vi "Cluster_AURA.vi"(0 "FOTOCELULA":bool, 1 "RFID_Error":errorcluster, 4 "RFID_LR6_Error":errorcluster, 6 "DC":bool, 7 "TEMPERATURA":bool, 8 "WHEEL_SENSOR":bool, 9 "all rows":dbl[][](array[numeric]), 10 "LIMITE MAX":dbl, 11 "LIMITE MIN":dbl, 12 "ERROR FPGA":errorcluster, 13 "ERROR ESCRITURA":errorcluster) -> (20 "appended array":cluster{string, dbl, "output string":string}[](array[cluster]), 22 "ESTADO WRD":dbl)   [LabVIEW 2015]
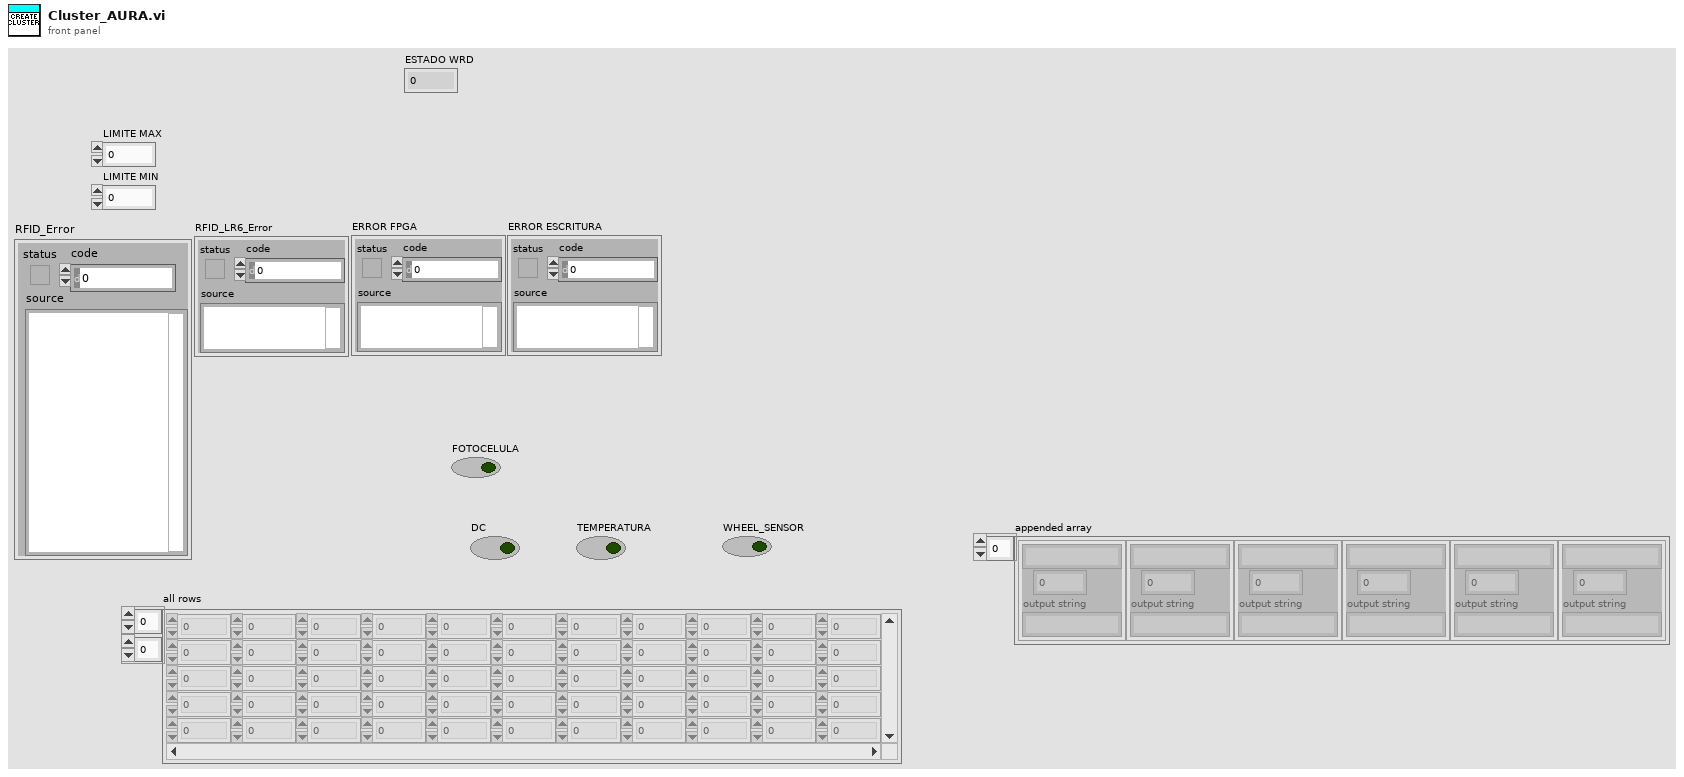
[diagram p1: front panel]
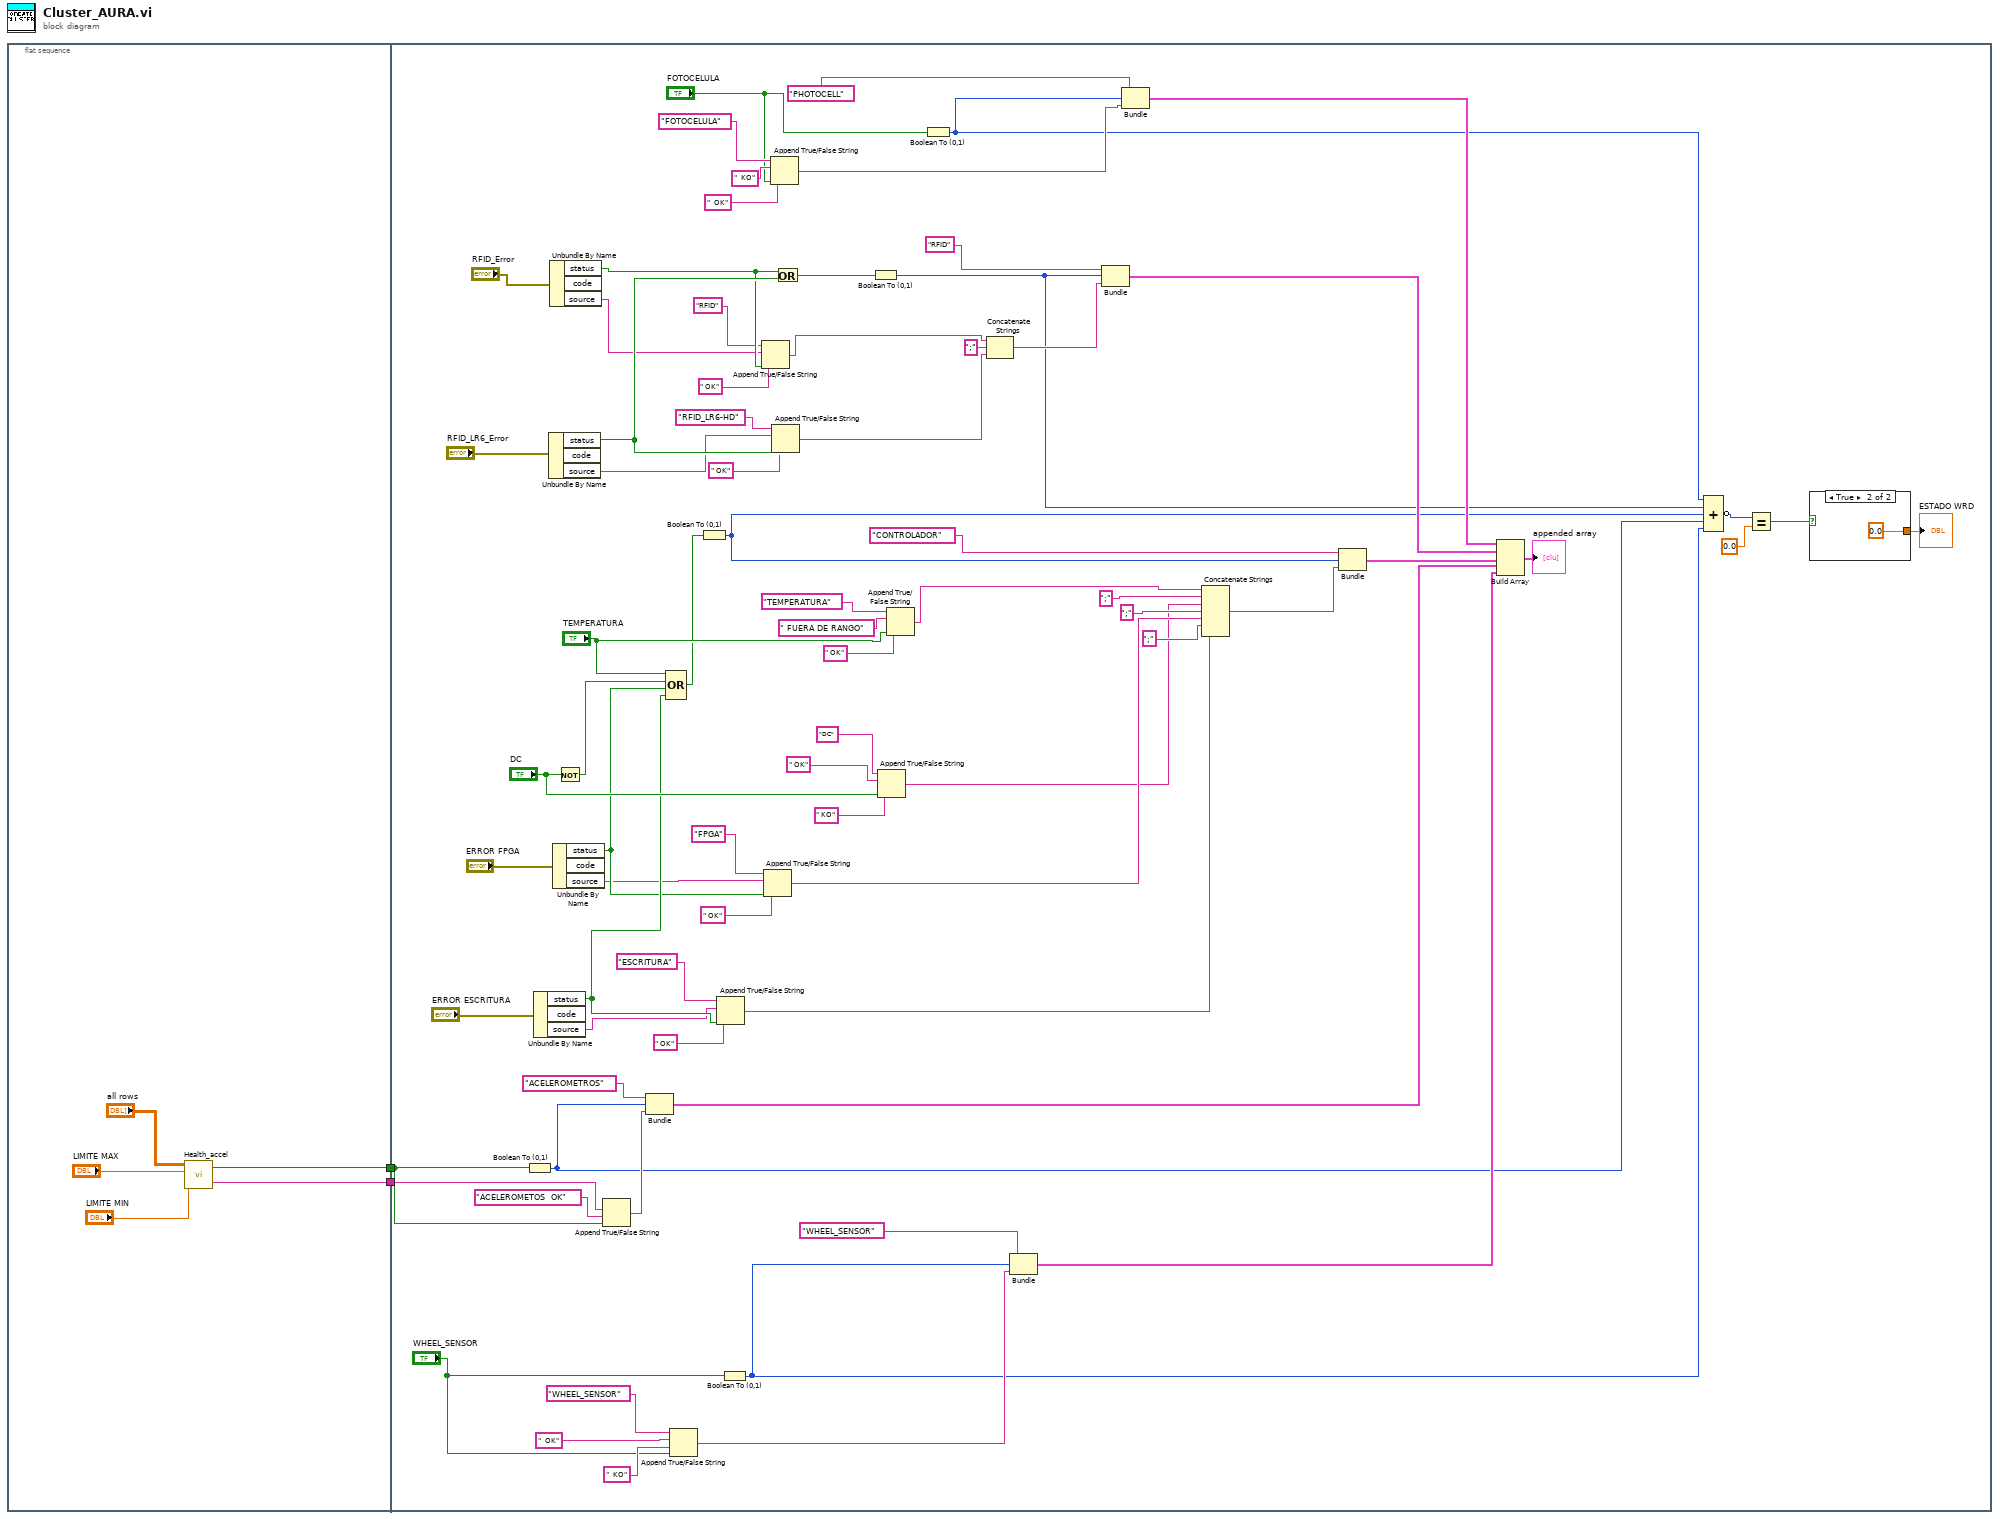
[diagram p0: block diagram]
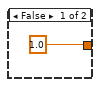
[diagram p2: hidden frame]
diagram:
  n1 = flat-sequence {
    tunnel: [w6] -> w2
    tunnel: [w5] -> w1
    tunnel: w2 -> [w31]
    tunnel: w1 -> [w11]
    frame #0 {
      n2 = call "Health_accel.vi"("LIMITE MIN"="LIMITE MIN", "LIMITE MAX"="LIMITE MAX", "Aceleraciones"="all rows") -> ("concatenated string"=w6:string, "ACELEROMETROS OK"=w5:bool)  [unwired: 3 in]
    }
    frame #1 {
      n3 = Boolean To (0,1)(Boolean=w11) -> (0, 1=w10:i16)
      n4 = Unbundle By Name("ERROR ESCRITURA") -> ("status"=w22:bool, "source"=w21:string)  [unwired: 1 out]
      n5 = Unbundle By Name("RFID_LR6_Error") -> ("status"=w72:bool, "source"=w26:string)  [unwired: 1 out]
      n6 = Unbundle By Name("RFID_Error") -> ("status"=w71:bool, "source"=w27:string)  [unwired: 1 out]
      n7 = Unbundle By Name("ERROR FPGA") -> ("status"=w19:bool, "source"=w18:string)  [unwired: 1 out]
      n8 = Not(x="DC") -> (.not. x?=w84:bool)
      n9 = Append True/False String(1:w11, 2:"ACELEROMETOS  OK" ("true string"), 3:w31) -> (0:w45:string)  [unwired: 1 in]
      n10 = Bundle("ACELEROMETROS", w10, "output string"=w45) -> (w51:cluster{string, i16, "output string":string})  [unwired: 1 in]
      n11 = Compound Arithmetic op=OR("TEMPERATURA", w84, w19, w22) -> (w13:bool)
      n12 = Append True/False String(1:"WHEEL_SENSOR", 2:"  KO" ("false string"), 3:"  OK" ("true string"), 4:"WHEEL_SENSOR" ("string (\"\")")) -> (0:w50:string)
      n13 = Boolean To (0,1)(Boolean=w13) -> (0, 1=w12:i16)
      n14 = Append True/False String(1:w22, 2:" OK" ("false string"), 3:w21, 4:"ESCRITURA" ("string (\"\")")) -> (0:w82:string)
      n15 = Boolean To (0,1)(Boolean="WHEEL_SENSOR") -> (0, 1=w8:i16)
      n16 = Append True/False String(1:w71, 2:" OK" ("false string"), 3:w27, 4:"RFID" ("string (\"\")")) -> (0:w60:string)
      n17 = Append True/False String(1:w19, 2:" OK" ("false string"), 3:w18, 4:"FPGA" ("string (\"\")")) -> (0:w80:string)
      n18 = Append True/False String(1:"FOTOCELULA", 2:"  OK" ("false string"), 3:"  KO" ("true string"), 4:"FOTOCELULA" ("string (\"\")")) -> (0:w35:string)
      n19 = Append True/False String(1:w72, 2:" OK" ("false string"), 3:w26, 4:"RFID_LR6-HD" ("string (\"\")")) -> (0:w75:string)
      n20 = Or(x=w71, y=w72) -> (x .or. y?=w15:bool)
      n21 = Boolean To (0,1)(Boolean=w15) -> (0, 1=w14:i16)
      n22 = Append True/False String(1:"DC", 2:" KO" ("false string"), 3:" OK" ("true string"), 4:"DC" ("string (\"\")")) -> (0:w78:string)
      n23 = Append True/False String(1:"TEMPERATURA", 2:" OK" ("false string"), 3:" FUERA DE RANGO" ("true string"), 4:"TEMPERATURA" ("string (\"\")")) -> (0:w66:string)
      n24 = Boolean To (0,1)(Boolean="FOTOCELULA") -> (0, 1=w16:i16)
      n25 = Concatenate Strings(w60, ";" ("string"), w75) -> (w61:string)
      n26 = Bundle("WHEEL_SENSOR", w8, "output string"=w50) -> (w52:cluster{string, i16, "output string":string})  [unwired: 1 in]
      n27 = Bundle("RFID", w14, w61) -> (w43:cluster{string, i16, string})  [unwired: 1 in]
      n28 = Bundle("PHOTOCELL", w16, "output string"=w35) -> (w34:cluster{string, i16, "output string":string})  [unwired: 1 in]
      n29 = Concatenate Strings(w66, ";", w78, ";", w80, ";", w82) -> (w67:string)
      n30 = Bundle("CONTROLADOR", w12, w67) -> (w58:cluster{string, i16, string})  [unwired: 1 in]
      n31 = Build Array(w34, w43, w58, w51, w52) -> (→"appended array":cluster{string, i16, "output string":string}[])
      n32 = Compound Arithmetic op=ADD(w16, w14, w12, w10, w8) -> (invert w30:i16)
      n33 = Equal?(x=w30, y=0.0) -> (x = y?=w28:bool)
      n34 = case shown="True" w28 {
        tunnel: [1.0 0.0] -> w73
        frame False {
        }
        frame True {
        }
      }
      "ESTADO WRD" <- w73
    }
  }
